vi "Replace Formula Variables.vi"(9 "Variables to be replaced":string[](array[string]), 11 "Formula in":string) -> (0 "Variables replaced?":bool, 1 "Formula variables":string[](array[string]), 3 "Formula out":string)   [LabVIEW 2020, in "Output Sequencer.lvlib" / "Settings UI.lvclass"]
uses:
  Settings UI.lvclass
  Output Sequencer/Output Sequencer.lvclass
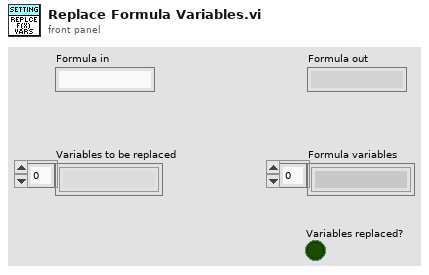
[diagram p1: front panel]
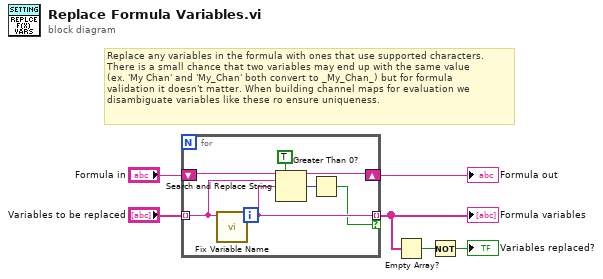
[diagram p0: block diagram]
diagram:
  # "Replace any variables in the formula with ones that use supported characters.\nThere is a small chance that two variables may end up with the same value\n(ex. 'My Chan' and 'My_Chan' both convert to _My_Chan_) but for formula\nvalidation it doesn't matter. When building channel maps for evaluation we\ndisambiguate variables like these ro ensure uniqueness."
  n1 = for {
    tunnel: "Variables to be replaced" -> [w11] mode=indexing
    tunnel: [w10] -> w3 mode=indexing if=w9
    shift-right: [w12] -> w6
    shift-left: "Formula in" -> [w13]
    n2 = call "Fix Variable Name.vi"("Variable in"=w11) -> ("Variable out"=w10:string)  [unwired: 10 in]
    n3 = Search and Replace String(replace all?=TRUE ("replace all? (F)"), input string=w13, search string=w11, replace string=w10) -> (result string=w12:string, number of replacements=w7:i32)  [unwired: 4 in, 2 out]
    n4 = Greater Than 0?(x=w7) -> (x > 0?=w9:bool)
  }
  "Formula variables" <- w3
  "Formula out" <- w6
  n5 = Empty Array?(array=w3) -> (empty?=w1:bool)
  n6 = Not(x=w1) -> (.not. x?=→"Variables replaced?":bool)
